vi "MGCC_IsdCon_global1.vi"() -> ()   [LabVIEW 2016]
doc: "-----------------------------------------------------------------------------------------------------------------------\nCopyright <2019> <The University of Tennessee at Knoxville and the University of Tennessee Research Foundation>\nThis software is released under BSD-3 \nhttps://opensource.org/licenses/BSD-3-Clause \nAdditional license options available at https://utrf.tennessee.edu/industry/sample-agreements/\n-----------------------------------------------------------------------------------------------------------------------"
panel:
  out "Planned_cleared":bool
  out "G4":bool
  out "G1":bool
  out "Grid Interface":bool[](array[boolean])
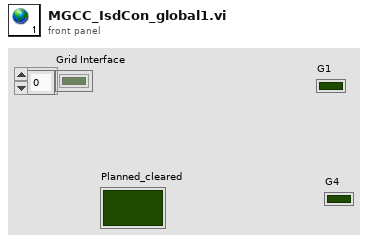
[diagram p1: front panel]
diagram:
